vi "JSON Request from Neural Network.vi"(11 "Features":dbl[](array[numeric])) -> (1 "t Delta":u32, 3 "x != 0?":bool)   [LabVIEW 2021]
uses:
  <vilib>/addons/_JKI.lib/REST Client/classes/REST Client/REST Client.lvclass
panel:
  out "Response body":string
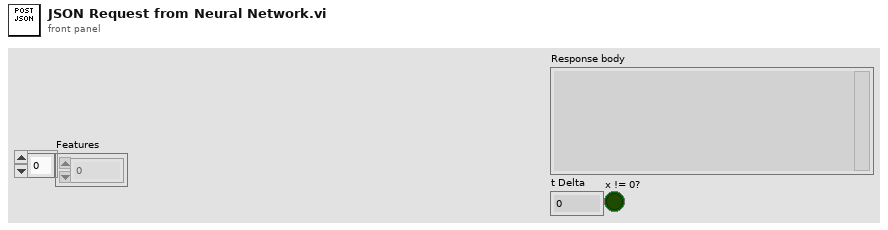
[diagram p1: front panel]
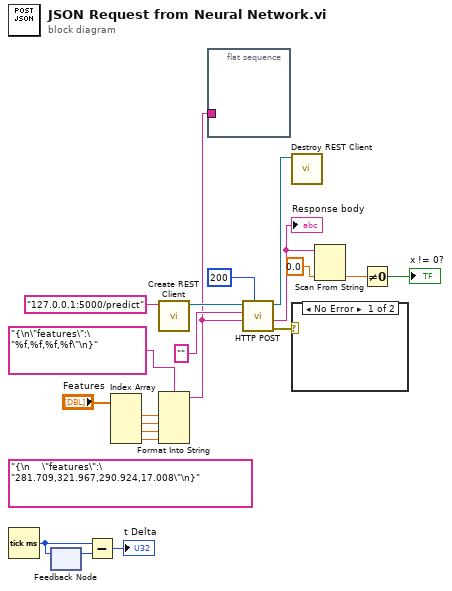
[diagram p0: block diagram]
diagram:
  (unwired) "{\n    \"features\":\"281.709,321.967,290.924,17.008\"\n}" ("Request body")
  n1 = Tick Count (ms)() -> (millisecond timer value=w17:u32)
  n2 = feedback-in #1(w17) -> ()
  n3 = feedback #1() -> (w16:u32)  [unwired: 1 in]
  n4 = Subtract(x=w17, y=w16) -> (x-y=→"t Delta":u32)
  n5 = Index Array(array="Features") -> (element #1=w4:dbl, element #2=w3:dbl, element #3=w2:dbl, element #4=w1:dbl)  [unwired: 4 in]
  n6 = call <vilib>:"Create REST Client.vi"("Base URL"="127.0.0.1:5000/predict") -> ("REST Client out"=w19:refnum<class "REST Client.lvclass">)  [unwired: 9 in, 1 out]
  n7 = Format Into String(format string="{\n\"features\":\"%f,%f,%f,%f\"\n}", w4, w3, w2, w1) -> (resulting string=w10:string)  [unwired: 2 in, 1 out]
  n8 = flat-sequence {
    tunnel: w10 -> [_]
    frame #0 {
    }
  }
  n9 = call-dynamic "HTTP POST.vi"("timeout (0 = Use Default)"=200, "Request body"=w10, "Path"="", "REST Client in"=w19) -> ("error out"=w13:errorcluster, "Response body"=w9:string, "REST Client out"=w14:refnum<class "REST Client.lvclass">)  [unwired: 2 in, 3 out]
  "Response body" <- w9
  n10 = call-dynamic "Destroy REST Client.vi"("REST Client in"=w14) -> ()  [unwired: 10 in, 1 out]
  n11 = case shown="No Error" w13 {
    frame No Error {
    }
    frame Error {
    }
  }
  n12 = Scan From String(input string=w9, default 1=0.0 ("default value 1")) -> (output 1=w7:dbl)  [unwired: 3 in, 3 out]
  n13 = Not Equal To 0?(x=w7) -> (x != 0?=→"x != 0?":bool)
